vi "log_acquisition.vi"(1 "log_data":T1) -> (0 "Log":string)   [LabVIEW 2017]
uses:
  log_data.ctl
  log_status.ctl
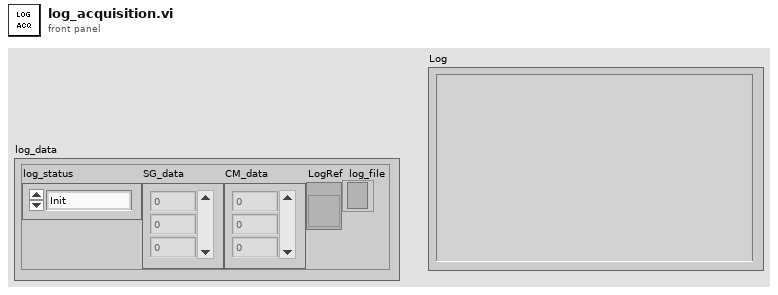
[diagram p1: front panel]
types:
  T1 = typedef "log_data.ctl" = cluster{"log_status":T2, "SG_data":dbl[], "CM_data":dbl[], "LogRef":refnum<vi>, "log_file":refnum<file>}
  T2 = typedef "log_status.ctl" = enum16{"Init", "Ready", "Running", "Error", "End"}
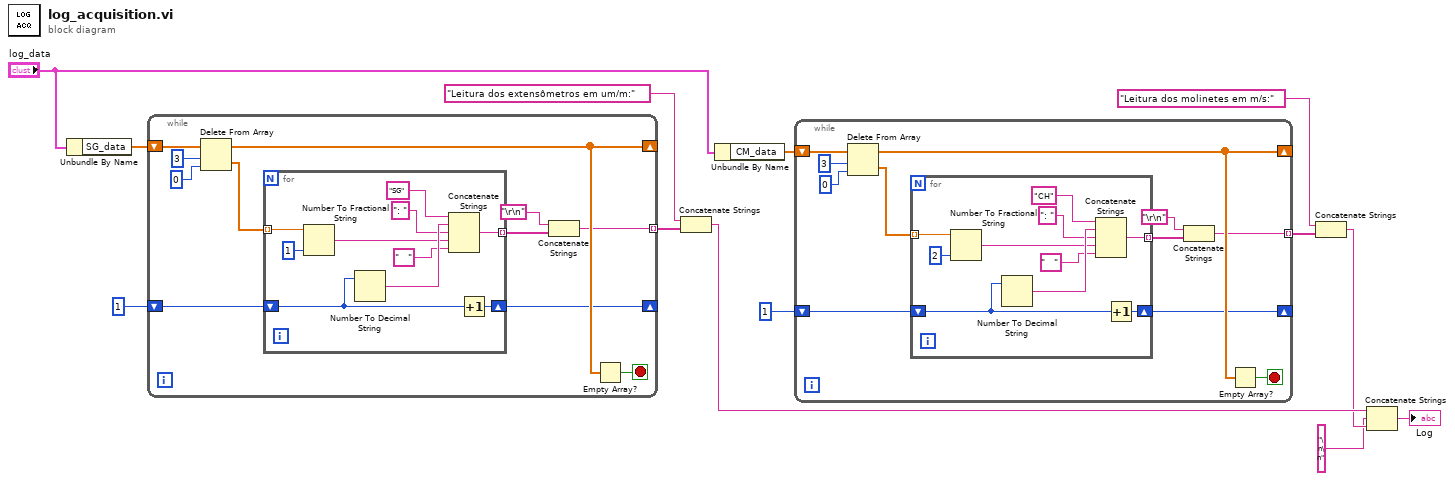
[diagram p0: block diagram]
diagram:
  n1 = Unbundle By Name("log_data") -> ("SG_data"=w13:dbl[])
  n2 = while {
    shift-right: [w21] -> _
    shift-left: w13 -> [w24]
    shift-right: [w17] -> _
    shift-left: i16 1 ("precision (6)") -> [w18]
    tunnel: [w14] -> w11 mode=indexing
    stop <- w20 stop-if-true
    n3 = Delete From Array(array=w24, length=3, index=0) -> (deleted portion=w19:dbl[], array with subset deleted=w21:dbl[])
    n4 = for {
      tunnel: w19 -> [w34] mode=indexing
      shift-right: [w32] -> w17
      shift-left: w18 -> [w31]
      tunnel: [w25] -> w16 mode=indexing
      n5 = Number To Fractional String(number=w34, precision (6)=i16 1) -> (F-format string=w27:string)  [unwired: 2 in]
      n6 = Number To Decimal String(number=w31) -> (decimal integer string=w30:string)  [unwired: 1 in]
      n7 = Concatenate Strings("SG" ("string"), w30, ": " ("string"), w27, "   " ("string")) -> (w25:string)
      n8 = Increment(x=w31) -> (x+1=w32:i16)
    }
    n9 = Concatenate Strings("\r\n", w16) -> (w14:string)
    n10 = Empty Array?(array=w21) -> (empty?=w20:bool)
  }
  n11 = Concatenate Strings("Leitura dos extensômetros em um/m:" ("string"), w11) -> (w4:string)
  n12 = Unbundle By Name("log_data") -> ("CM_data"=w6:dbl[])
  n13 = while {
    shift-right: [w42] -> _
    shift-left: w6 -> [w45]
    shift-right: [w38] -> _
    shift-left: i16 1 ("precision (6)") -> [w39]
    tunnel: [w35] -> w8 mode=indexing
    stop <- w41 stop-if-true
    n14 = Delete From Array(array=w45, length=3, index=0) -> (deleted portion=w40:dbl[], array with subset deleted=w42:dbl[])
    n15 = for {
      tunnel: w40 -> [w55] mode=indexing
      shift-right: [w53] -> w38
      shift-left: w39 -> [w52]
      tunnel: [w46] -> w37 mode=indexing
      n16 = Number To Fractional String(number=w55, precision (6)=i16 2) -> (F-format string=w48:string)  [unwired: 2 in]
      n17 = Number To Decimal String(number=w52) -> (decimal integer string=w51:string)  [unwired: 1 in]
      n18 = Concatenate Strings("CH" ("string"), w51, ": " ("string"), w48, "   " ("string")) -> (w46:string)
      n19 = Increment(x=w52) -> (x+1=w53:i16)
    }
    n20 = Concatenate Strings("\r\n", w37) -> (w35:string)
    n21 = Empty Array?(array=w42) -> (empty?=w41:bool)
  }
  n22 = Concatenate Strings("Leitura dos molinetes em m/s:" ("string"), w8) -> (w2:string)
  n23 = Concatenate Strings(w4, "\n\n" ("string"), w2) -> (→"Log":string)
